vi "Verify.vi"(8 "error in":errorcluster, 10 "original file path":path, 11 "new file path":path) -> (0 "error out":errorcluster, 3 "new file path out":path)   [LabVIEW 2023]
doc: "Validate the correctness of the newly created TDMS file."
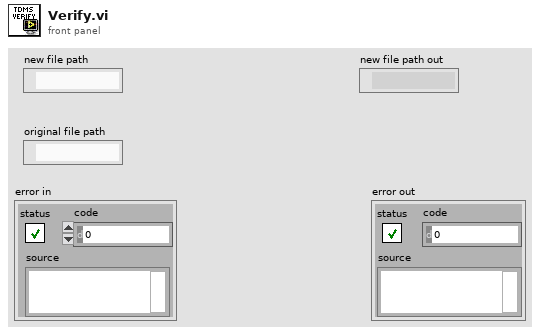
[diagram p1: front panel]
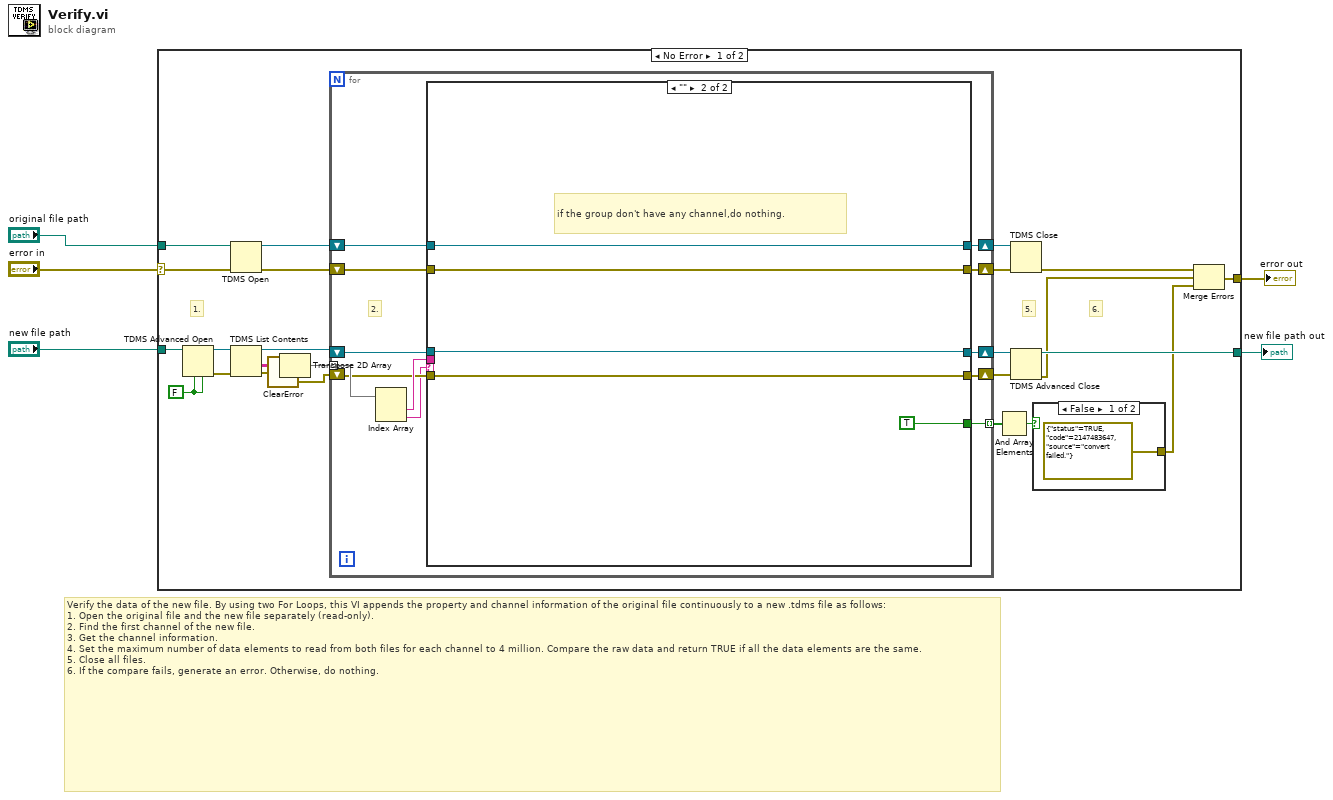
[diagram p0: block diagram]
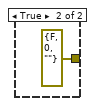
[diagram p2: hidden frame]
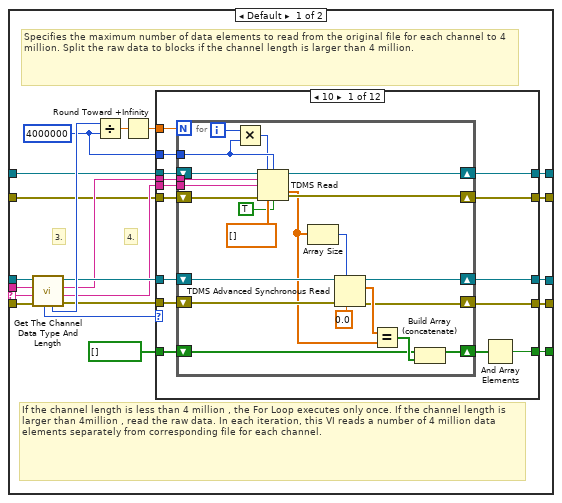
[diagram p3: hidden frame]
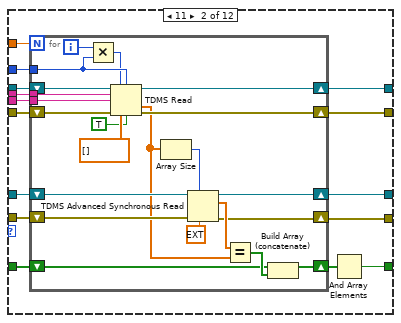
[diagram p4: hidden frame]
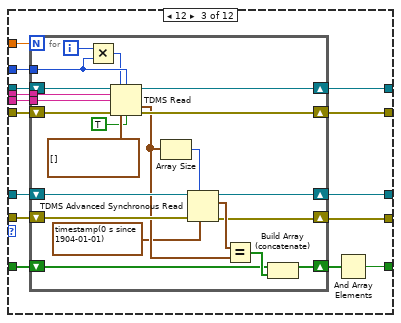
[diagram p5: hidden frame]
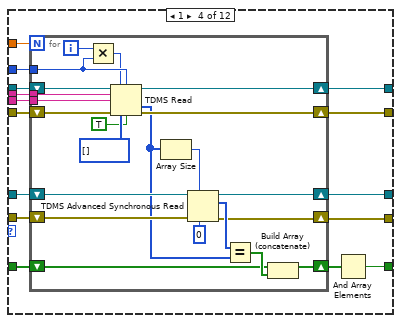
[diagram p6: hidden frame]
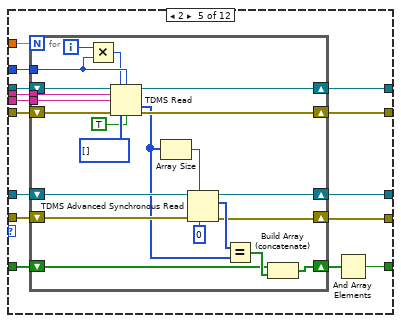
[diagram p7: hidden frame]
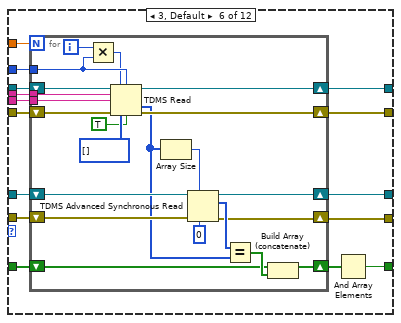
[diagram p8: hidden frame]
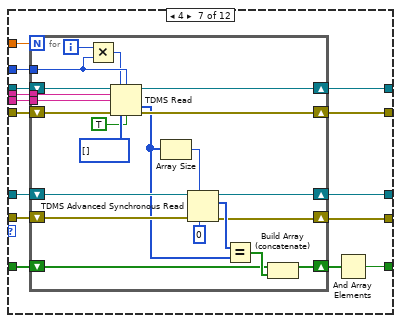
[diagram p9: hidden frame]
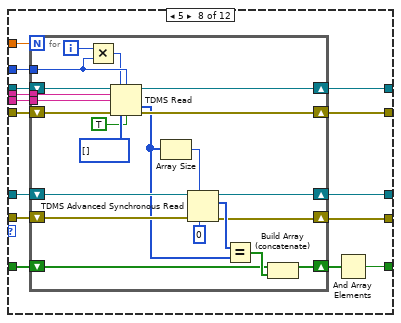
[diagram p10: hidden frame]
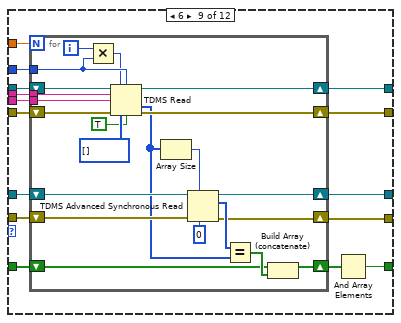
[diagram p11: hidden frame]
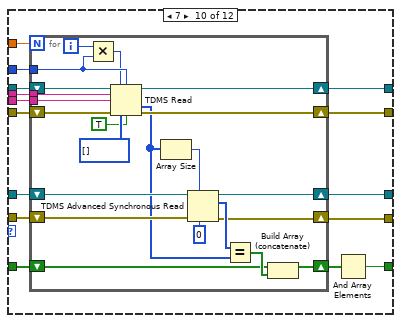
[diagram p12: hidden frame]
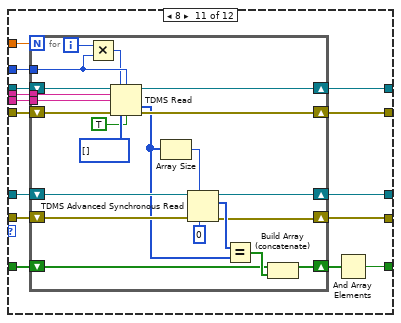
[diagram p13: hidden frame]
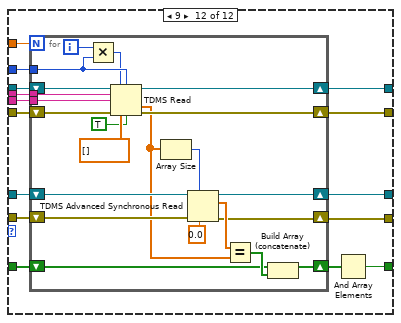
[diagram p14: hidden frame]
diagram:
  # "Verify the data of the new file. By using two For Loops, this VI appends the property and channel information of the original file continuously to a new .tdms file as follows:\n1. Open the original file and the new file separately (read-only).\n2. Find the first channel of the new file.\n3. Get the channel information.\n4. Set the maximum number of data elements to read from both files for each channel to 4 million. Compare the raw data and return TRUE if all the data elements are the same.\n5. Close all files.\n6. If the compare fails, generate an error. Otherwise, do nothing."
  n1 = case shown="No Error" "error in" {
    selector: "error in" -> [w23 w515]
    tunnel: [w29 w514] -> w5
    tunnel: [w8 w515] -> w4
    tunnel: "new file path" -> [w25 w514]
    tunnel: "original file path" -> [w24 _]
    frame No Error {
      w7 = FALSE ("enable asynchronous? (T)")
      # "6."
      # "5."
      # "1."
      n2 = TDMS Advanced Open(4:w7, 6:w7, 11:w25) -> (0:w18:errorcluster, 3:w20:refnum<k34>)  [unwired: 2 in, 1 out]
      n3 = TDMS Open(8:w23, 11:w24) -> (0:w15:errorcluster, 3:w22:refnum<k34>)  [unwired: 5 in]
      n4 = TDMS List Contents(4:w18, 7:w20) -> (0:w6:errorcluster, 1:w21:string[][], 3:w19:refnum<k34>)  [unwired: 1 in, 1 out]
      n5 = call <vilib>:"ClearError.vi"("error in (no error)"=w6) -> ("error out"=w17:errorcluster)
      n6 = Transpose 2D Array(2D array=w21) -> (transposed array=w16:string[][])
      n7 = for {
        shift-right: [w42] -> w14
        shift-left: w22 -> [w43]
        shift-right: [w39] -> w12
        shift-left: w19 -> [w33]
        shift-right: [w41] -> w13
        shift-left: w15 -> [w35]
        tunnel: [w40] -> w28 mode=indexing
        shift-right: [w38] -> w11
        shift-left: w17 -> [w34]
        tunnel: w16 -> [w37] mode=indexing
        # "2."
        n8 = Index Array(array=w37) -> (element #1=w36:string, element #2=w32:string)  [unwired: 2 in]
        n9 = case shown="\"\"" w32 {
          selector: w32 -> [w62 _]
          tunnel: w43 -> [w51 w513]
          tunnel: [w57 w509] -> w39
          tunnel: [w54 w513] -> w42
          tunnel: w35 -> [w47 w512]
          tunnel: [w59 w512] -> w41
          tunnel: [w55 TRUE] -> w40
          tunnel: [w53 w510] -> w38
          tunnel: w36 -> [w50 _]
          tunnel: w34 -> [w46 w510]
          tunnel: w33 -> [w45 w509]
          frame Default {
            w61 = 4000000 ("y")
            # "If the channel length is less than 4 million , the For Loop executes only once. If the channel length is larger than 4million , read the raw data. In each iteration, this VI reads a number of 4 million data elements separately from corresponding file for each channel."
            # "Specifies the maximum number of data elements to read from the original file for each channel to 4 million. Split the raw data to blocks if the channel length is larger than 4 million."
            # "4."
            # "3."
            n10 = call "Get The Channel Data Type And Length.vi"("error in (no error)"=w46, "channel name"=w62, "group name"=w50, "tdms file"=w45) -> ("error out"=w44:errorcluster, "dup channel name"=w48:string, "dup group name"=w49:string, "dup tdms file"=w52:refnum<k34>, "channel length"=w64:i32, "data type"=w60:i32)  [unwired: 2 in]
            n11 = Divide(x=w64, y=w61) -> (x/y=w63:dbl)
            n12 = Round Toward +Infinity(x=w63) -> (ceil(x): smallest int >= x=w58:dbl)
            n13 = case shown="10" w60 {
              tunnel: w61 -> [w77 w114 w151 w188 w225 w262 w299 w336 w373 w410 w447 w484]
              tunnel: w52 -> [w79 w116 w153 w190 w227 w264 w301 w338 w375 w412 w449 w486]
              tunnel: [w71 w108 w145 w182 w219 w256 w293 w330 w367 w404 w441 w478] -> w57
              tunnel: [w74 w111 w148 w185 w222 w259 w296 w333 w370 w407 w444 w481] -> w59
              tunnel: w51 -> [w78 w115 w152 w189 w226 w263 w300 w337 w374 w411 w448 w485]
              tunnel: w47 -> [w73 w110 w147 w184 w221 w258 w295 w332 w369 w406 w443 w480]
              tunnel: w49 -> [w76 w113 w150 w187 w224 w261 w298 w335 w372 w409 w446 w483]
              tunnel: w48 -> [w75 w112 w149 w186 w223 w260 w297 w334 w371 w408 w445 w482]
              tunnel: w58 -> [w72 w109 w146 w183 w220 w257 w294 w331 w368 w405 w442 w479]
              tunnel: bool[] [] -> [w70 w107 w144 w181 w218 w255 w292 w329 w366 w403 w440 w477]
              tunnel: [w68 w105 w142 w179 w216 w253 w290 w327 w364 w401 w438 w475] -> w55
              tunnel: [w67 w104 w141 w178 w215 w252 w289 w326 w363 w400 w437 w474] -> w54
              tunnel: w44 -> [w66 w103 w140 w177 w214 w251 w288 w325 w362 w399 w436 w473]
              tunnel: [w65 w102 w139 w176 w213 w250 w287 w324 w361 w398 w435 w472] -> w53
              frame 10 {
                n14 = for {
                  N: w72 -> [_]
                  tunnel: w77 -> [w92]
                  tunnel: w76 -> [w95]
                  tunnel: w75 -> [w94]
                  shift-right: [w85] -> w74
                  shift-left: w73 -> [w90]
                  shift-right: [w100] -> w71
                  shift-left: w79 -> [w101]
                  shift-right: [w86] -> w67
                  shift-left: w78 -> [w99]
                  shift-right: [w88] -> w69
                  shift-left: w70 -> [w87]
                  shift-right: [w83] -> w65
                  shift-left: w66 -> [w84]
                  i -> [w93]
                  n15 = Multiply(x=w93, y=w92) -> (x*y=w91:i32)
                  n16 = TDMS Read(0:w99, 1:w91, 2:w92, 5:w95, 7:w94, 11:w90, 12:dbl[] [], 13:TRUE ("return channels in file order? (F)")) -> (4:w86:refnum<k34>, 10:w82:dbl[], 15:w85:errorcluster)  [unwired: 3 out]
                  n17 = Array Size(array=w82) -> (size(s)=w81:i32)
                  n18 = TDMS Advanced Synchronous Read(6:0.0 ("U64"), 7:w81, 8:w84, 11:w101) -> (0:w83:errorcluster, 2:w97:dbl[], 3:w100:refnum<k34>)  [unwired: 1 out]
                  n19 = Equal?(x=w97, y=w82) -> (x = y?=w89:bool[])
                  n20 = Build Array (concatenate)(w87, w89) -> (w88:bool[])
                }
                n21 = And Array Elements(Boolean array=w69) -> (logical AND=w68:bool)
              }
              frame 11 {
                n22 = for {
                  N: w109 -> [_]
                  tunnel: w114 -> [w129]
                  tunnel: w113 -> [w132]
                  tunnel: w112 -> [w131]
                  shift-right: [w122] -> w111
                  shift-left: w110 -> [w127]
                  shift-right: [w137] -> w108
                  shift-left: w116 -> [w138]
                  shift-right: [w123] -> w104
                  shift-left: w115 -> [w136]
                  shift-right: [w125] -> w106
                  shift-left: w107 -> [w124]
                  shift-right: [w120] -> w102
                  shift-left: w103 -> [w121]
                  i -> [w130]
                  n23 = Multiply(x=w130, y=w129) -> (x*y=w128:i32)
                  n24 = TDMS Read(0:w136, 1:w128, 2:w129, 5:w132, 7:w131, 11:w127, 12:ext[] [], 13:TRUE ("return channels in file order? (F)")) -> (4:w123:refnum<k34>, 10:w119:ext[], 15:w122:errorcluster)  [unwired: 3 out]
                  n25 = Array Size(array=w119) -> (size(s)=w118:i32)
                  n26 = TDMS Advanced Synchronous Read(6:ext 0.0 ("U64"), 7:w118, 8:w121, 11:w138) -> (0:w120:errorcluster, 2:w134:ext[], 3:w137:refnum<k34>)  [unwired: 1 out]
                  n27 = Equal?(x=w134, y=w119) -> (x = y?=w126:bool[])
                  n28 = Build Array (concatenate)(w124, w126) -> (w125:bool[])
                }
                n29 = And Array Elements(Boolean array=w106) -> (logical AND=w105:bool)
              }
              frame 12 {
                n30 = for {
                  N: w146 -> [_]
                  tunnel: w151 -> [w168]
                  tunnel: w150 -> [w171]
                  tunnel: w149 -> [w170]
                  shift-right: [w161] -> w148
                  shift-left: w147 -> [w166]
                  shift-right: [w174] -> w145
                  shift-left: w153 -> [w175]
                  shift-right: [w162] -> w141
                  shift-left: w152 -> [w173]
                  shift-right: [w164] -> w143
                  shift-left: w144 -> [w163]
                  shift-right: [w159] -> w139
                  shift-left: w140 -> [w160]
                  i -> [w169]
                  n31 = Multiply(x=w169, y=w168) -> (x*y=w167:i32)
                  n32 = TDMS Read(0:w173, 1:w167, 2:w168, 5:w171, 7:w170, 11:w166, 12:timestamp[] [], 13:TRUE ("return channels in file order? (F)")) -> (4:w162:refnum<k34>, 10:w158:timestamp[], 15:w161:errorcluster)  [unwired: 3 out]
                  n33 = Array Size(array=w158) -> (size(s)=w157:i32)
                  n34 = TDMS Advanced Synchronous Read(6:timestamp(0 s since 1904-01-01), 7:w157, 8:w160, 11:w175) -> (0:w159:errorcluster, 2:w172:timestamp[], 3:w174:refnum<k34>)  [unwired: 1 out]
                  n35 = Equal?(x=w172, y=w158) -> (x = y?=w165:bool[])
                  n36 = Build Array (concatenate)(w163, w165) -> (w164:bool[])
                }
                n37 = And Array Elements(Boolean array=w143) -> (logical AND=w142:bool)
              }
              frame 1 {
                n38 = for {
                  N: w183 -> [_]
                  tunnel: w188 -> [w203]
                  tunnel: w187 -> [w206]
                  tunnel: w186 -> [w205]
                  shift-right: [w196] -> w185
                  shift-left: w184 -> [w201]
                  shift-right: [w211] -> w182
                  shift-left: w190 -> [w212]
                  shift-right: [w197] -> w178
                  shift-left: w189 -> [w210]
                  shift-right: [w199] -> w180
                  shift-left: w181 -> [w198]
                  shift-right: [w194] -> w176
                  shift-left: w177 -> [w195]
                  i -> [w204]
                  n39 = Multiply(x=w204, y=w203) -> (x*y=w202:i32)
                  n40 = TDMS Read(0:w210, 1:w202, 2:w203, 5:w206, 7:w205, 11:w201, 12:i8[] [], 13:TRUE ("return channels in file order? (F)")) -> (4:w197:refnum<k34>, 10:w193:i8[], 15:w196:errorcluster)  [unwired: 3 out]
                  n41 = Array Size(array=w193) -> (size(s)=w192:i32)
                  n42 = TDMS Advanced Synchronous Read(6:i8 0 ("U64"), 7:w192, 8:w195, 11:w212) -> (0:w194:errorcluster, 2:w208:i8[], 3:w211:refnum<k34>)  [unwired: 1 out]
                  n43 = Equal?(x=w208, y=w193) -> (x = y?=w200:bool[])
                  n44 = Build Array (concatenate)(w198, w200) -> (w199:bool[])
                }
                n45 = And Array Elements(Boolean array=w180) -> (logical AND=w179:bool)
              }
              frame 2 {
                n46 = for {
                  N: w220 -> [_]
                  tunnel: w225 -> [w240]
                  tunnel: w224 -> [w243]
                  tunnel: w223 -> [w242]
                  shift-right: [w233] -> w222
                  shift-left: w221 -> [w238]
                  shift-right: [w248] -> w219
                  shift-left: w227 -> [w249]
                  shift-right: [w234] -> w215
                  shift-left: w226 -> [w247]
                  shift-right: [w236] -> w217
                  shift-left: w218 -> [w235]
                  shift-right: [w231] -> w213
                  shift-left: w214 -> [w232]
                  i -> [w241]
                  n47 = Multiply(x=w241, y=w240) -> (x*y=w239:i32)
                  n48 = TDMS Read(0:w247, 1:w239, 2:w240, 5:w243, 7:w242, 11:w238, 12:i16[] [], 13:TRUE ("return channels in file order? (F)")) -> (4:w234:refnum<k34>, 10:w230:i16[], 15:w233:errorcluster)  [unwired: 3 out]
                  n49 = Array Size(array=w230) -> (size(s)=w229:i32)
                  n50 = TDMS Advanced Synchronous Read(6:i16 0 ("U64"), 7:w229, 8:w232, 11:w249) -> (0:w231:errorcluster, 2:w245:i16[], 3:w248:refnum<k34>)  [unwired: 1 out]
                  n51 = Equal?(x=w245, y=w230) -> (x = y?=w237:bool[])
                  n52 = Build Array (concatenate)(w235, w237) -> (w236:bool[])
                }
                n53 = And Array Elements(Boolean array=w217) -> (logical AND=w216:bool)
              }
              frame 3, Default {
                n54 = for {
                  N: w257 -> [_]
                  tunnel: w262 -> [w277]
                  tunnel: w261 -> [w280]
                  tunnel: w260 -> [w279]
                  shift-right: [w270] -> w259
                  shift-left: w258 -> [w275]
                  shift-right: [w285] -> w256
                  shift-left: w264 -> [w286]
                  shift-right: [w271] -> w252
                  shift-left: w263 -> [w284]
                  shift-right: [w273] -> w254
                  shift-left: w255 -> [w272]
                  shift-right: [w268] -> w250
                  shift-left: w251 -> [w269]
                  i -> [w278]
                  n55 = Multiply(x=w278, y=w277) -> (x*y=w276:i32)
                  n56 = TDMS Read(0:w284, 1:w276, 2:w277, 5:w280, 7:w279, 11:w275, 12:i32[] [], 13:TRUE ("return channels in file order? (F)")) -> (4:w271:refnum<k34>, 10:w267:i32[], 15:w270:errorcluster)  [unwired: 3 out]
                  n57 = Array Size(array=w267) -> (size(s)=w266:i32)
                  n58 = TDMS Advanced Synchronous Read(6:0 ("U64"), 7:w266, 8:w269, 11:w286) -> (0:w268:errorcluster, 2:w282:i32[], 3:w285:refnum<k34>)  [unwired: 1 out]
                  n59 = Equal?(x=w282, y=w267) -> (x = y?=w274:bool[])
                  n60 = Build Array (concatenate)(w272, w274) -> (w273:bool[])
                }
                n61 = And Array Elements(Boolean array=w254) -> (logical AND=w253:bool)
              }
              frame 4 {
                n62 = for {
                  N: w294 -> [_]
                  tunnel: w299 -> [w314]
                  tunnel: w298 -> [w317]
                  tunnel: w297 -> [w316]
                  shift-right: [w307] -> w296
                  shift-left: w295 -> [w312]
                  shift-right: [w322] -> w293
                  shift-left: w301 -> [w323]
                  shift-right: [w308] -> w289
                  shift-left: w300 -> [w321]
                  shift-right: [w310] -> w291
                  shift-left: w292 -> [w309]
                  shift-right: [w305] -> w287
                  shift-left: w288 -> [w306]
                  i -> [w315]
                  n63 = Multiply(x=w315, y=w314) -> (x*y=w313:i32)
                  n64 = TDMS Read(0:w321, 1:w313, 2:w314, 5:w317, 7:w316, 11:w312, 12:i64[] [], 13:TRUE ("return channels in file order? (F)")) -> (4:w308:refnum<k34>, 10:w304:i64[], 15:w307:errorcluster)  [unwired: 3 out]
                  n65 = Array Size(array=w304) -> (size(s)=w303:i32)
                  n66 = TDMS Advanced Synchronous Read(6:i64 0 ("U64"), 7:w303, 8:w306, 11:w323) -> (0:w305:errorcluster, 2:w319:i64[], 3:w322:refnum<k34>)  [unwired: 1 out]
                  n67 = Equal?(x=w319, y=w304) -> (x = y?=w311:bool[])
                  n68 = Build Array (concatenate)(w309, w311) -> (w310:bool[])
                }
                n69 = And Array Elements(Boolean array=w291) -> (logical AND=w290:bool)
              }
              frame 5 {
                n70 = for {
                  N: w331 -> [_]
                  tunnel: w336 -> [w351]
                  tunnel: w335 -> [w354]
                  tunnel: w334 -> [w353]
                  shift-right: [w344] -> w333
                  shift-left: w332 -> [w349]
                  shift-right: [w359] -> w330
                  shift-left: w338 -> [w360]
                  shift-right: [w345] -> w326
                  shift-left: w337 -> [w358]
                  shift-right: [w347] -> w328
                  shift-left: w329 -> [w346]
                  shift-right: [w342] -> w324
                  shift-left: w325 -> [w343]
                  i -> [w352]
                  n71 = Multiply(x=w352, y=w351) -> (x*y=w350:i32)
                  n72 = TDMS Read(0:w358, 1:w350, 2:w351, 5:w354, 7:w353, 11:w349, 12:u8[] [], 13:TRUE ("return channels in file order? (F)")) -> (4:w345:refnum<k34>, 10:w341:u8[], 15:w344:errorcluster)  [unwired: 3 out]
                  n73 = Array Size(array=w341) -> (size(s)=w340:i32)
                  n74 = TDMS Advanced Synchronous Read(6:u8 0 ("U64"), 7:w340, 8:w343, 11:w360) -> (0:w342:errorcluster, 2:w356:u8[], 3:w359:refnum<k34>)  [unwired: 1 out]
                  n75 = Equal?(x=w356, y=w341) -> (x = y?=w348:bool[])
                  n76 = Build Array (concatenate)(w346, w348) -> (w347:bool[])
                }
                n77 = And Array Elements(Boolean array=w328) -> (logical AND=w327:bool)
              }
              frame 6 {
                n78 = for {
                  N: w368 -> [_]
                  tunnel: w373 -> [w388]
                  tunnel: w372 -> [w391]
                  tunnel: w371 -> [w390]
                  shift-right: [w381] -> w370
                  shift-left: w369 -> [w386]
                  shift-right: [w396] -> w367
                  shift-left: w375 -> [w397]
                  shift-right: [w382] -> w363
                  shift-left: w374 -> [w395]
                  shift-right: [w384] -> w365
                  shift-left: w366 -> [w383]
                  shift-right: [w379] -> w361
                  shift-left: w362 -> [w380]
                  i -> [w389]
                  n79 = Multiply(x=w389, y=w388) -> (x*y=w387:i32)
                  n80 = TDMS Read(0:w395, 1:w387, 2:w388, 5:w391, 7:w390, 11:w386, 12:u16[] [], 13:TRUE ("return channels in file order? (F)")) -> (4:w382:refnum<k34>, 10:w378:u16[], 15:w381:errorcluster)  [unwired: 3 out]
                  n81 = Array Size(array=w378) -> (size(s)=w377:i32)
                  n82 = TDMS Advanced Synchronous Read(6:u16 0 ("U64"), 7:w377, 8:w380, 11:w397) -> (0:w379:errorcluster, 2:w393:u16[], 3:w396:refnum<k34>)  [unwired: 1 out]
                  n83 = Equal?(x=w393, y=w378) -> (x = y?=w385:bool[])
                  n84 = Build Array (concatenate)(w383, w385) -> (w384:bool[])
                }
                n85 = And Array Elements(Boolean array=w365) -> (logical AND=w364:bool)
              }
              frame 7 {
                n86 = for {
                  N: w405 -> [_]
                  tunnel: w410 -> [w425]
                  tunnel: w409 -> [w428]
                  tunnel: w408 -> [w427]
                  shift-right: [w418] -> w407
                  shift-left: w406 -> [w423]
                  shift-right: [w433] -> w404
                  shift-left: w412 -> [w434]
                  shift-right: [w419] -> w400
                  shift-left: w411 -> [w432]
                  shift-right: [w421] -> w402
                  shift-left: w403 -> [w420]
                  shift-right: [w416] -> w398
                  shift-left: w399 -> [w417]
                  i -> [w426]
                  n87 = Multiply(x=w426, y=w425) -> (x*y=w424:i32)
                  n88 = TDMS Read(0:w432, 1:w424, 2:w425, 5:w428, 7:w427, 11:w423, 12:u32[] [], 13:TRUE ("return channels in file order? (F)")) -> (4:w419:refnum<k34>, 10:w415:u32[], 15:w418:errorcluster)  [unwired: 3 out]
                  n89 = Array Size(array=w415) -> (size(s)=w414:i32)
                  n90 = TDMS Advanced Synchronous Read(6:u32 0 ("U64"), 7:w414, 8:w417, 11:w434) -> (0:w416:errorcluster, 2:w430:u32[], 3:w433:refnum<k34>)  [unwired: 1 out]
                  n91 = Equal?(x=w430, y=w415) -> (x = y?=w422:bool[])
                  n92 = Build Array (concatenate)(w420, w422) -> (w421:bool[])
                }
                n93 = And Array Elements(Boolean array=w402) -> (logical AND=w401:bool)
              }
              frame 8 {
                n94 = for {
                  N: w442 -> [_]
                  tunnel: w447 -> [w462]
                  tunnel: w446 -> [w465]
                  tunnel: w445 -> [w464]
                  shift-right: [w455] -> w444
                  shift-left: w443 -> [w460]
                  shift-right: [w470] -> w441
                  shift-left: w449 -> [w471]
                  shift-right: [w456] -> w437
                  shift-left: w448 -> [w469]
                  shift-right: [w458] -> w439
                  shift-left: w440 -> [w457]
                  shift-right: [w453] -> w435
                  shift-left: w436 -> [w454]
                  i -> [w463]
                  n95 = Multiply(x=w463, y=w462) -> (x*y=w461:i32)
                  n96 = TDMS Read(0:w469, 1:w461, 2:w462, 5:w465, 7:w464, 11:w460, 12:u64[] [], 13:TRUE ("return channels in file order? (F)")) -> (4:w456:refnum<k34>, 10:w452:u64[], 15:w455:errorcluster)  [unwired: 3 out]
                  n97 = Array Size(array=w452) -> (size(s)=w451:i32)
                  n98 = TDMS Advanced Synchronous Read(6:u64 0 ("U64"), 7:w451, 8:w454, 11:w471) -> (0:w453:errorcluster, 2:w467:u64[], 3:w470:refnum<k34>)  [unwired: 1 out]
                  n99 = Equal?(x=w467, y=w452) -> (x = y?=w459:bool[])
                  n100 = Build Array (concatenate)(w457, w459) -> (w458:bool[])
                }
                n101 = And Array Elements(Boolean array=w439) -> (logical AND=w438:bool)
              }
              frame 9 {
                n102 = for {
                  N: w479 -> [_]
                  tunnel: w484 -> [w499]
                  tunnel: w483 -> [w502]
                  tunnel: w482 -> [w501]
                  shift-right: [w492] -> w481
                  shift-left: w480 -> [w497]
                  shift-right: [w507] -> w478
                  shift-left: w486 -> [w508]
                  shift-right: [w493] -> w474
                  shift-left: w485 -> [w506]
                  shift-right: [w495] -> w476
                  shift-left: w477 -> [w494]
                  shift-right: [w490] -> w472
                  shift-left: w473 -> [w491]
                  i -> [w500]
                  n103 = Multiply(x=w500, y=w499) -> (x*y=w498:i32)
                  n104 = TDMS Read(0:w506, 1:w498, 2:w499, 5:w502, 7:w501, 11:w497, 12:sgl[] [], 13:TRUE ("return channels in file order? (F)")) -> (4:w493:refnum<k34>, 10:w489:sgl[], 15:w492:errorcluster)  [unwired: 3 out]
                  n105 = Array Size(array=w489) -> (size(s)=w488:i32)
                  n106 = TDMS Advanced Synchronous Read(6:sgl 0.0 ("U64"), 7:w488, 8:w491, 11:w508) -> (0:w490:errorcluster, 2:w504:sgl[], 3:w507:refnum<k34>)  [unwired: 1 out]
                  n107 = Equal?(x=w504, y=w489) -> (x = y?=w496:bool[])
                  n108 = Build Array (concatenate)(w494, w496) -> (w495:bool[])
                }
                n109 = And Array Elements(Boolean array=w476) -> (logical AND=w475:bool)
              }
            }
          }
          frame "" {
            # "if the group don't have any channel,do nothing."
          }
        }
      }
      n110 = And Array Elements(Boolean array=w28) -> (logical AND=w10:bool)
      n111 = TDMS Close(8:w13, 11:w14) -> (0:w27:errorcluster)  [unwired: 1 out]
      n112 = TDMS Advanced Close(8:w11, 11:w12) -> (0:w26:errorcluster, 3:w29:path)  [unwired: 2 in]
      n113 = case shown="False" w10 {
        tunnel: [errorcluster {"status"=TRUE, "code"=2147483647, "source"="convert failed."} ("error in") errorcluster {"status"=FALSE, "code"=0, "source"=""} ("error in")] -> w9
        frame False {
        }
        frame True {
        }
      }
      n114 = Merge Errors(w27, w26, w9) -> (w8:errorcluster)
    }
    frame Error {
    }
  }
  "error out" <- w4
  "new file path out" <- w5
